vi "Rx Section Page.vi"(8 "error in (no error)":errorcluster, 11 "Node Ptr":T1 format="%.0x") -> (0 "error out":errorcluster)   [LabVIEW 2016, in "UDP-Custom-Device System Explorer.lvlib"]
uses:
  UDP-Custom-Device System Explorer.lvlib
  <vilib>/NI Veristand/Custom Device API/Custom Device Item Ref.ctl
  Types/TypeDef - Rx Section Page References.ctl
  Shared/Constants.vi
  <vilib>/NI Veristand/Custom Device API/Set Item Property (I32 Array).vi
  <vilib>/NI VeriStand/Custom Device API/Custom Device API.lvlib
  Shared/UDP-Custom-Device Shared.lvlib
panel:
  in  "Rx Packets":i32[](listbox)
  in  "SHDocVw.IWebBrowser":refnum<k7>(container)
  in  "General Header":cluster{"Section Name":string}={"Section Name"="Configured Packets"}
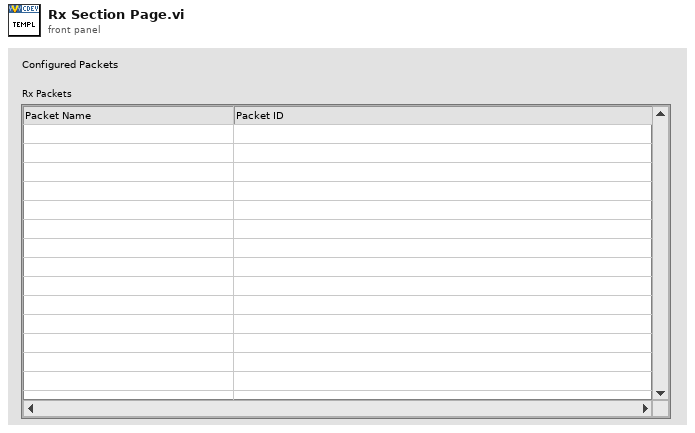
[diagram p1: front panel]
types:
  T1 = typedef "Custom Device API.lvlib/Custom Device Item Ref.ctl" = u64
  T2 = typedef "UDP-Custom-Device System Explorer.lvlib/TypeDef - Rx Section Page References.ctl" = cluster{"Name":refnum<vi>, "Description":refnum<vi>, "Rx Packets":refnum<vi>, "Auto Assign Local NIC?":refnum<vi>, "IP Address of Local NIC":refnum<vi>, "Port":refnum<vi>, "Packet ID":refnum<vi>}
  T3 = typedef "Custom Device API.lvlib/Custom Device Commands.ctl" = enum16{"Default", "Item renamed", "Shutdown", "Dynamic button pressed"}
  T4 = typedef "LVPoint32TypeDef.ctl" = cluster{"Horizontal":i32, "Vertical":i32}
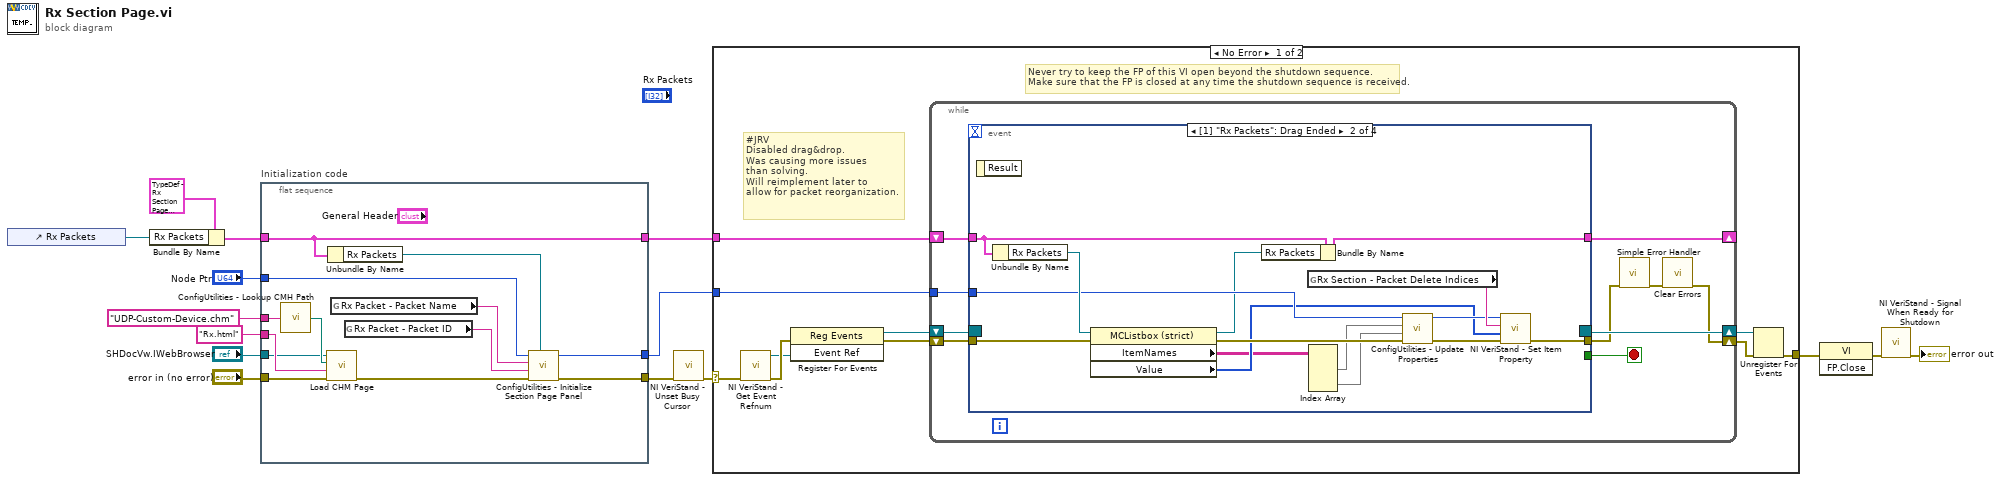
[diagram p0: block diagram]
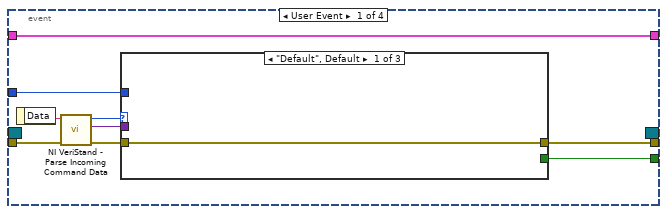
[diagram p2: hidden frame]
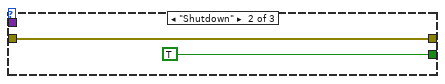
[diagram p3: hidden frame]
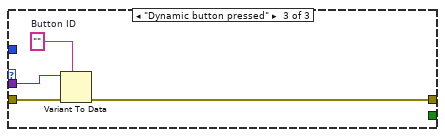
[diagram p4: hidden frame]
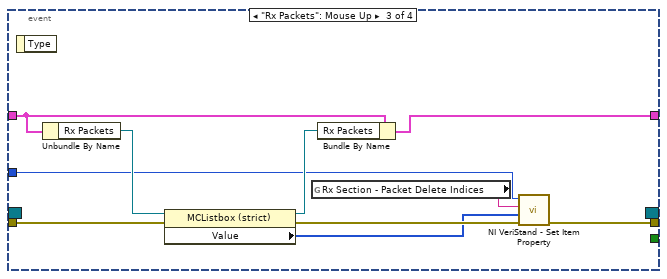
[diagram p5: hidden frame]
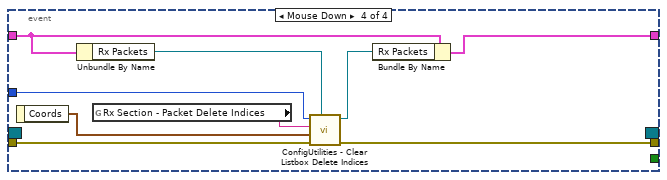
[diagram p6: hidden frame]
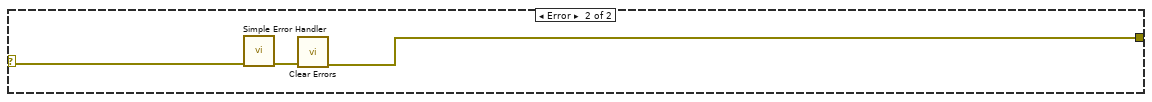
[diagram p7: hidden frame]
diagram:
  n1 = control-ref of="Rx Packets"() -> (w5:refnum<vi>)
  n2 = Bundle By Name(cluster=T2 {"Name"=refnum, "Description"=refnum, "Rx Packets"=refnum, "Auto Assign Local NIC?"=refnum, "IP Address of Local NIC"=refnum, "Port"=refnum, "Packet ID"=refnum} ("Rx Section Cluster"), "Rx Packets"=w5) -> (w4:T2)
  n3 = flat-sequence "Initialization code" {
    tunnel: "error in (no error)" -> [w20]
    tunnel: "Node Ptr" -> [w26]
    tunnel: [w27] -> w12
    tunnel: [w25] -> w9
    tunnel: "SHDocVw.IWebBrowser" -> [w17]
    tunnel: "Rx.html" ("CD_CHM_Section") -> [w18]
    tunnel: "UDP-Custom-Device.chm" ("CD_CHM_FileName") -> [w19]
    tunnel: w4 -> [w28]
    tunnel: [w28] -> w3
    frame #0 {
      n4 = call "ConfigUtilities - Lookup CMH Path.vi"("Main CMH File"=w19) -> ("Compiled CMH Path"=w21:path)
      n5 = call <vilib>:"Load CHM Page.vi"("error in (no error)"=w20, "HTML File"=w18, "Compiled CHM Path"=w21, "Web Browser Reference"=w17) -> ("error out"=w16:errorcluster)  [unwired: 7 in]
      n6 = Unbundle By Name(w28) -> ("Rx Packets"=w22:refnum<vi>)
      n7 = global read "Constants.vi" "Rx Packet - Packet Name"() -> (w24:string)
      n8 = global read "Constants.vi" "Rx Packet - Packet ID"() -> (w23:string)
      n9 = call "ConfigUtilities - Initialize Section Page Panel.vi"("Packets Listbox"=w22, "error in (no error)"=w16, "Packet IDs Property"=w23, "Packet Names Property"=w24, "Item Ref in"=w26) -> ("error out"=w27:errorcluster, "Item Ref out"=w25:T1)  [unwired: 3 in, 2 out]
    }
  }
  n10 = call <vilib>:"NI VeriStand - Unset Busy Cursor.vi"("error in (no error)"=w12) -> ("error out"=w11:errorcluster)  [unwired: 10 out]
  n11 = case shown="No Error" w11 {
    selector: w11 -> [w30 w101]
    tunnel: [w35 w99] -> w15
    tunnel: w9 -> [w31 _]
    tunnel: w3 -> [w29 _]
    frame No Error {
      # "#JRV\nDisabled drag&drop.\nWas causing more issues\nthan solving.\nWill reimplement later to\nallow for packet reorganization."
      # "Never try to keep the FP of this VI open beyond the shutdown sequence.\nMake sure that the FP is closed at any time the shutdown sequence is received."
      n12 = call <vilib>:"NI VeriStand - Get Event Refnum.vi"("error in (no error)"=w30) -> ("error out"=w38:errorcluster, "Event Ref"=w34:refnum<user-event>)  [unwired: 9 out]
      n13 = register-events(error in=w38, w34) -> (reference out=w32:refnum<event-registration>, error out=w33:errorcluster)  [unwired: 1 in]
      n14 = while {
        tunnel: w31 -> [w44]
        shift-right: [w41] -> w36
        shift-left: w33 -> [w47]
        shift-right: [w48] -> w37
        shift-left: w32 -> [w46]
        shift-right: [w39] -> _
        shift-left: w29 -> [w40]
        stop <- w45 stop-if-true
        n15 = event shown="[1] \"Rx Packets\": Drag Ended" {
          selector: w46 -> [_ _ _ _]
          dyn-events: [_ _ _ _] -> w48
          timeout: _ -> [_ _ _ _]
          tunnel: w47 -> [w57 w79 w89 w98]
          tunnel: [w53 _ _ _] -> w45
          tunnel: [w52 w75 w84 w90] -> w43
          tunnel: w44 -> [w51 w72 w80 w96]
          tunnel: w40 -> [w49 w67 w83 w92]
          tunnel: [w49 w66 w82 w93] -> w39
          event User Event {
            n16 = event-data() -> ("Data"=w56:string)  [unwired: 1 out]
            n17 = call <vilib>:"NI VeriStand - Parse Incoming Command Data.vi"("error in (no error)"=w57, "Incoming data"=w56) -> ("error out"=w55:errorcluster, "Outgoing data"=w50:variant, "Action"=w54:T3)  [unwired: 7 out]
            n18 = case shown="\"Default\", Default" w54 {
              tunnel: w55 -> [w58 w59 w64]
              tunnel: [_ TRUE _] -> w53
              tunnel: [w58 w59 w61] -> w52
              tunnel: w51 -> [_ _ _]
              tunnel: w50 -> [_ _ w63]
              frame "Default", Default {
              }
              frame "Shutdown" {
              }
              frame "Dynamic button pressed" {
                w62 = ""  # Button ID
                n19 = Variant To Data(error in=w64, type=w62, Variant=w63) -> (error out=w61:errorcluster)  [unwired: 1 out]
              }
            }
          }
          event "Rx Packets": Drag Ended {
            n20 = event-data() -> ()  [unwired: 2 out]
            n21 = Unbundle By Name(w67) -> ("Rx Packets"=w78:refnum<vi>)
            n22 = property class="MCListbox (strict)"(reference=w78, error in=w79) -> (reference out=w65:refnum<vi>, error out=w77:errorcluster, "ItemNames"=w70:string[][], "Value"=w71:i32[])
            n23 = Bundle By Name(cluster=w67, "Rx Packets"=w65) -> (w66:T2)
            n24 = global read "Constants.vi" "Rx Section - Packet Delete Indices"() -> (w74:string)
            n25 = Index Array(array=w70) -> (element #1=w69:string[], element #2=w68:string[])  [unwired: 4 in]
            n26 = call "ConfigUtilities - Update Properties.vi"("error in (no error)"=w77, "Channel Paths"=w68, "Channel Names"=w69, "Item Ref in"=w72) -> ("error out"=w76:errorcluster, "Item Ref out"=w73:T1)  [unwired: 6 in]
            n27 = call-poly <vilib>:"NI VeriStand - Set Item Property.vi"("error in (no error)"=w76, "Value"=w71, "Property Name"=w74, "Item Ref in"=w73) -> ("error out"=w75:errorcluster)  [unwired: 5 in, 2 out]
          }
          event "Rx Packets": Mouse Up {
            n28 = event-data() -> ()  [unwired: 2 out]
            n29 = Unbundle By Name(w83) -> ("Rx Packets"=w88:refnum<vi>)
            n30 = property class="MCListbox (strict)"(reference=w88, error in=w89) -> (reference out=w81:refnum<vi>, error out=w87:errorcluster, "Value"=w86:i32[])
            n31 = global read "Constants.vi" "Rx Section - Packet Delete Indices"() -> (w85:string)
            n32 = Bundle By Name(cluster=w83, "Rx Packets"=w81) -> (w82:T2)
            n33 = call-poly <vilib>:"NI VeriStand - Set Item Property.vi"("error in (no error)"=w87, "Value"=w86, "Property Name"=w85, "Item Ref in"=w80) -> ("error out"=w84:errorcluster)  [unwired: 5 in, 2 out]
          }
          event Mouse Down {
            n34 = event-data() -> ("Coords"=w97:T4)  [unwired: 1 out]
            n35 = Unbundle By Name(w92) -> ("Rx Packets"=w91:refnum<vi>)
            n36 = global read "Constants.vi" "Rx Section - Packet Delete Indices"() -> (w95:string)
            n37 = call "ConfigUtilities - Clear Listbox Delete Indices.vi"("Listbox Reference in"=w91, "error in (no error)"=w98, "Pane Coords"=w97, "Delete Property Name"=w95, "Item Ref in"=w96) -> ("error out"=w90:errorcluster, "Listbox Reference out"=w94:refnum<vi>)  [unwired: 5 in]
            n38 = Bundle By Name(cluster=w92, "Rx Packets"=w94) -> (w93:T2)
          }
        }
        n39 = call <vilib>:"Simple Error Handler.vi"("error in (no error)"=w43) -> ("error out"=w42:errorcluster)  [unwired: 1 in, 7 out]
        n40 = call <vilib>:"Clear Errors.vi"("error in (no error)"=w42) -> ("error out"=w41:errorcluster)  [unwired: 1 in, 5 out]
      }
      n41 = Unregister For Events(event registration refnum=w37, error in=w36) -> (error out=w35:errorcluster)
    }
    frame Error {
      n42 = call <vilib>:"Simple Error Handler.vi"("error in (no error)"=w101) -> ("error out"=w100:errorcluster)  [unwired: 1 in, 7 out]
      n43 = call <vilib>:"Clear Errors.vi"("error in (no error)"=w100) -> ("error out"=w99:errorcluster)  [unwired: 1 in, 5 out]
    }
  }
  n44 = invoke class="VI" method="FP.Close"(error in=w15) -> (error out=w14:errorcluster)  [unwired: 2 in, 2 out]
  n45 = call <vilib>:"NI VeriStand - Signal When Ready for Shutdown.vi"("error in (no error)"=w14) -> ("error out"=→"error out":errorcluster)  [unwired: 10 out]
